vi "GR_Servo.vi"() -> ()   [LabVIEW 2015]
panel:
  out "RPT DATA 2":string[][](array[string])
  out "RPT DATA":string[][](array[string])
  out "Load DATA":dbl
  in  "Error Message":string
  out "STM Done Bit LCD Pressing":bool
  in  "Direction M2":bool
  in  "Servo On Bit M 2":bool
  in  "Mode M2":i32(ring)=10178 items=["Finite Samples"=10178, "Continuous Samples"=10123, "Hardware Timed Single Point"=12522]
  in  "Speed d/s M2":i32=10
  in  "Travel (Degree) M2":i32=100
  in  "Direction M1":bool
  in  "Servo On Bit M1":bool
  in  "ModeM1":i32(ring)=10178 items=["Finite Samples"=10178, "Continuous Samples"=10123, "Hardware Timed Single Point"=12522]
  in  "Speed d/s M1":i32=10
  in  "Travel (Degree)M1":i32=100
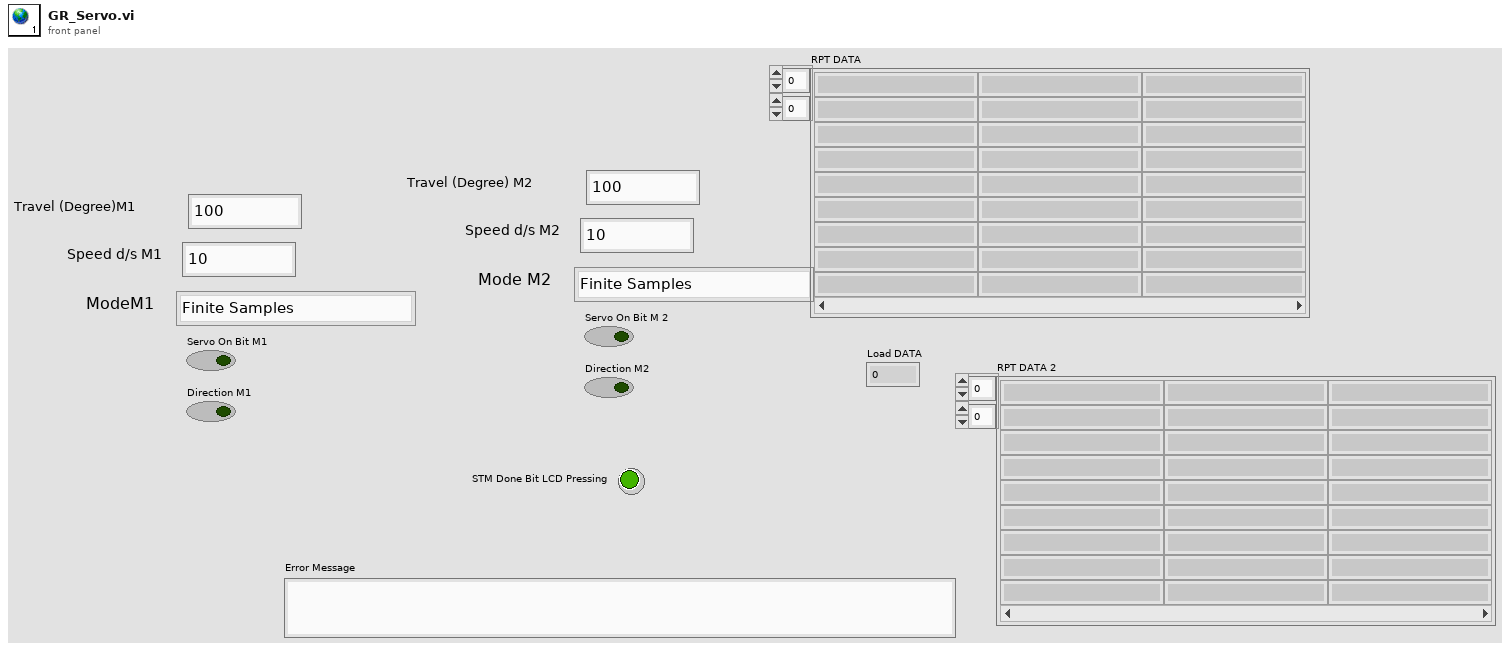
[diagram p1: front panel]
diagram:
